vi "set32bitInteger.vi"(11 "inI32":i32) -> ()   [LabVIEW 2014]
uses:
  GlobalVariables.vi
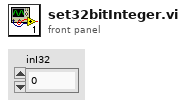
[diagram p1: front panel]
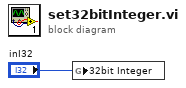
[diagram p0: block diagram]
diagram:
  n1 = global write "GlobalVariables.vi" "32bit Integer"("inI32") -> ()
